vi "Image Initialization.vi"(1 "Image Names":u16(ring) items=["Image", "Template", "Edge"], 8 "error in":errorcluster, 10 "Image Definition":T3(array[cluster])=[{"Border Size"=3, "Image Name"="Image", "Image Type"=5}, {"Border Size"=3, "Image Name"="Template", "Image Type"=5}, {"Border Size"=3, "Image Name"="Edge", "Image Type"=0}] {"Image Type" items=["Grayscale (U8)", "Grayscale (I16)", "Grayscale (SGL)", "Complex (CSG)", "RGB (U32)", "HSL (U32)", "RGB (U64)", "Grayscale (U16)"]}) -> (0 "error out":errorcluster, 2 "Images":T1[](array[typedef]))   [LabVIEW 2014]
uses:
  <vilib>/vision/Image Controls.llb/IMAQ Image.ctl
  <vilib>/Utility/miscctls.llb/LVStringsAndValuesArrayTypeDef.ctl
panel:
  # "LICENSED MATERIALS – PROPERTY OF IBM\nCopyright IBM Corp. 2016,\nALL RIGHTS RESERVED"
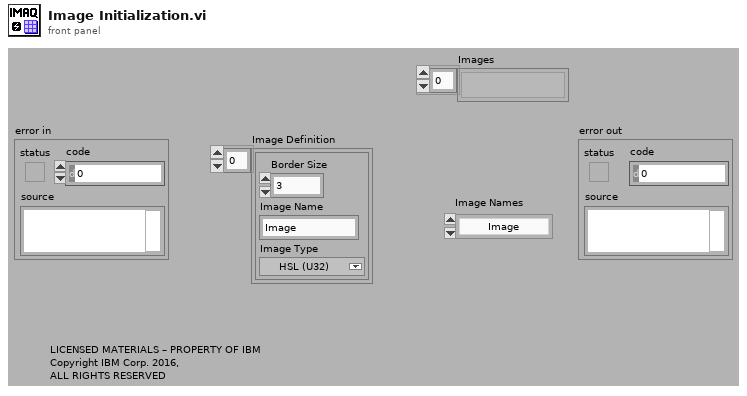
[diagram p1: front panel]
types:
  T1 = typedef "IMAQ Image.ctl" = refnum<image>
  T2 = typedef "Image Type" = u32
  T3 = cluster{"Border Size":i32, "Image Name":string, "Image Type":T2}[]
  T4 = typedef "LVStringsAndValuesArrayTypeDef.ctl" = cluster{"String":string, "Value":ext}[]
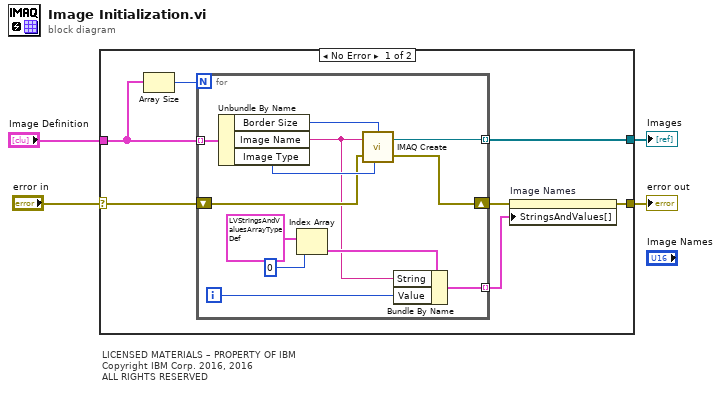
[diagram p0: block diagram]
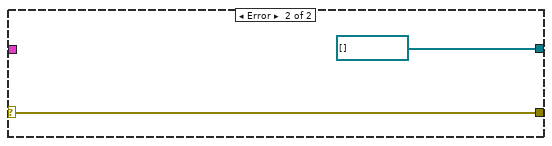
[diagram p2: hidden frame]
diagram:
  # "LICENSED MATERIALS – PROPERTY OF IBM\nCopyright IBM Corp. 2016, 2016\nALL RIGHTS RESERVED"
  n1 = case shown="No Error" "error in" {
    selector: "error in" -> [w10 w25]
    tunnel: "Image Definition" -> [w9 _]
    tunnel: [w11 T1[] []] -> w3
    tunnel: [w5 w25] -> w1
    frame No Error {
      n2 = Array Size(array=w9) -> (size(s)=w8:i32)
      n3 = for {
        N: w8 -> [_]
        tunnel: w9 -> [w23] mode=indexing
        tunnel: [w20] -> w11 mode=indexing
        shift-right: [w18] -> w6
        shift-left: w10 -> [w19]
        tunnel: [w12] -> w7 mode=indexing
        i -> [w14]
        n4 = Unbundle By Name(w23) -> ("Border Size"=w22:i32, "Image Name"=w13:string, "Image Type"=w21:T2)
        n5 = Index Array(array=T4 [{"String"="", "Value"=0.0}] ("Strings And Values []"), index=0) -> (element=w15:cluster{"String":string, "Value":ext})
        n6 = call "IMAQ Create"("Border Size"=w22, "Image Name"=w13, "Image Type"=w21, "error in (no error)"=w19) -> ("New Image"=w20:T1, "error out"=w18:errorcluster)  [unwired: 1 out]
        n7 = Bundle By Name(cluster=w15, "String"=w13, "Value"=w14) -> (w12:cluster{"String":string, "Value":ext})
      }
      n8 = property on="Image Names" class="Ring (strict)"(error in=w6, "StringsAndValues[]"=w7) -> (error out=w5:errorcluster)  [unwired: 1 in, 1 out]
    }
    frame Error {
    }
  }
  "Images" <- w3
  "error out" <- w1
